vi "Process Channel.vi"(0 "Software Lock-in in":refnum<class "Software Lock-in.lvclass">, 1 "tdms file":refnum<k34>, 2 "Phase":dbl, 5 "Group name":string, 9 "Channel name":string, 11 "error in (no error)":errorcluster, 12 "Time constant":dbl, 13 "Harmonic":i32=1) -> (3 "tdms file out":refnum<k34>, 4 "Software Lock-in out":refnum<class "Software Lock-in.lvclass">, 6 "Signal":dynamicdata(graph), 7 "found":bool, 8 "Time axis":dbl[](array[numeric]), 10 "Channel names":string[](array[string]), 14 "dt":dbl, 15 "error out":errorcluster)   [LabVIEW 2020, in "Software Lock-in.lvclass"]
uses:
  Software Lock-in.lvclass
  C:/GitHub/NHMFL_Core/Libraries/SoftwareLockin/Lock-in Detector/Lock-in Detector.lvclass
  Software Lock-in.lvclass/Software Lock-in.ctl
  Lock-in Detector/Lock-in Detector.lvclass/Lock-in Detector.ctl
  Lock-in Detector/Read Reference phase.vi
  Lock-in Detector/Write Reference phase.vi
  Lock-in Detector/Write Harmonic.vi
  Lock-in Detector/Write Time constant.vi
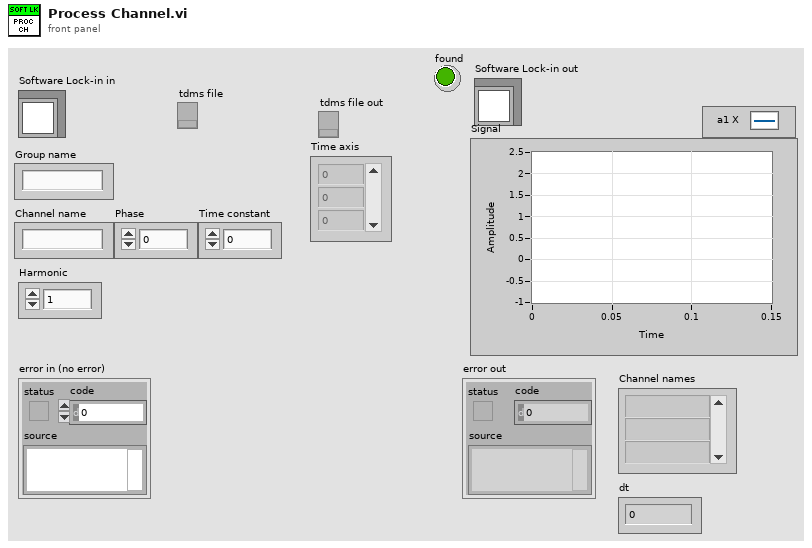
[diagram p1: front panel]
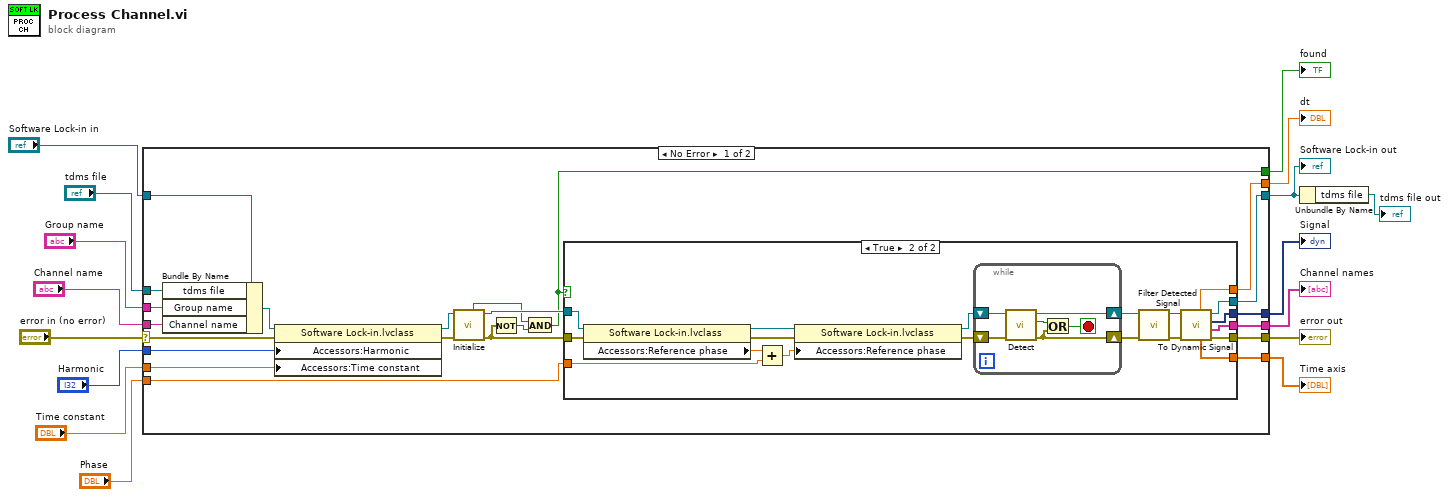
[diagram p0: block diagram]
diagram:
  n1 = case shown="No Error" "error in (no error)" {
    selector: "error in (no error)" -> [w37 w67]
    tunnel: [w34 w67] -> w15
    tunnel: [w35 w66] -> w13
    tunnel: "Software Lock-in in" -> [w38 w66]
    tunnel: "Harmonic" -> [w18 _]
    tunnel: "Channel name" -> [w33 _]
    tunnel: "Group name" -> [w32 _]
    tunnel: "Time constant" -> [w17 _]
    tunnel: "tdms file" -> [w31 _]
    tunnel: [w30 _] -> w6
    tunnel: [w29 _] -> w5
    tunnel: [w28 _] -> w4
    tunnel: [w27 _] -> w3
    tunnel: "Phase" -> [w26 _]
    tunnel: [w22 _] -> w1
    frame No Error {
      n2 = Bundle By Name(cluster=w38, "tdms file"=w31, "Group name"=w32, "Channel name"=w33) -> (w20:refnum<class "Software Lock-in.lvclass">)
      n3 = property class="Software Lock-in.lvclass"(reference=w20, error in=w37, "Accessors:Harmonic"=w18, "Accessors:Time constant"=w17) -> (reference out=w19:refnum<class "Software Lock-in.lvclass">, error out=w21:errorcluster)
      n4 = call-dynamic "Initialize.vi"("error in (no error)"=w21, "Software Lock-in in"=w19) -> ("error out"=w24:errorcluster, "Software Lock-in out"=w36:refnum<class "Software Lock-in.lvclass">, "found"=w25:bool)  [unwired: 7 in]
      n5 = Not(x=w24) -> (.not. x?=w23:bool)
      n6 = And(x=w25, y=w23) -> (x .and. y?=w22:bool)
      n7 = case shown="True" w22 {
        tunnel: w24 -> [w40 w59]
        tunnel: w36 -> [w39 w46]
        tunnel: [w39 w55] -> w35
        tunnel: [w40 w53] -> w34
        tunnel: [_ w52] -> w30
        tunnel: [_ w51] -> w29
        tunnel: [_ w50] -> w28
        tunnel: [_ w49] -> w27
        tunnel: w26 -> [_ w48]
        frame False {
        }
        frame True {
          n8 = property class="Software Lock-in.lvclass"(reference=w46, error in=w59) -> (reference out=w45:refnum<class "Software Lock-in.lvclass">, error out=w47:errorcluster, "Accessors:Reference phase"=w44:dbl)
          n9 = Add(x=w44, y=w48) -> (x+y=w41:dbl)
          n10 = property class="Software Lock-in.lvclass"(reference=w45, error in=w47, "Accessors:Reference phase"=w41) -> (reference out=w42:refnum<class "Software Lock-in.lvclass">, error out=w43:errorcluster)
          n11 = while {
            shift-right: [w63] -> w58
            shift-left: w42 -> [w65]
            shift-right: [w60] -> w57
            shift-left: w43 -> [w62]
            stop <- w61 stop-if-true
            n12 = call-dynamic "Detect.vi"("error in (no error)"=w62, "Software Lock-in in"=w65) -> ("error out"=w60:errorcluster, "Finished"=w64:bool, "Software Lock-in out"=w63:refnum<class "Software Lock-in.lvclass">)  [unwired: 7 in]
            n13 = Or(x=w64, y=w60) -> (x .or. y?=w61:bool)
          }
          n14 = call-dynamic "Filter Detected Signal.vi"("error in (no error)"=w57, "Software Lock-in in"=w58) -> ("error out"=w54:errorcluster, "Software Lock-in out"=w56:refnum<class "Software Lock-in.lvclass">)  [unwired: 8 in]
          n15 = call "To Dynamic Signal.vi"("error in (no error)"=w54, "Software Lock-in in"=w56) -> ("error out"=w53:errorcluster, "Channel names"=w50:string[], "Signal"=w49:dynamicdata, "Software Lock-in out"=w55:refnum<class "Software Lock-in.lvclass">, "Time axis"=w51:dbl[], "dt"=w52:dbl)  [unwired: 4 in]
        }
      }
    }
    frame Error {
    }
  }
  "error out" <- w15
  "Software Lock-in out" <- w13
  "dt" <- w6
  "Time axis" <- w5
  "Channel names" <- w4
  "Signal" <- w3
  "found" <- w1
  n16 = Unbundle By Name(w13) -> ("tdms file"=→"tdms file out":refnum<k34>)
